vi "Read Name.vi"(8 "error in (no error)":errorcluster, 11 "Player in":refnum<class "Player.lvclass">) -> (0 "error out":errorcluster, 2 "Name":u16(ring) items=["玩家1", "玩家2"], 3 "Player out":refnum<class "Player.lvclass">)   [LabVIEW 2009, in "Player.lvclass"]
doc: "Get the name of the current player."
uses:
  Player.lvclass
  Player.lvclass/Player.ctl
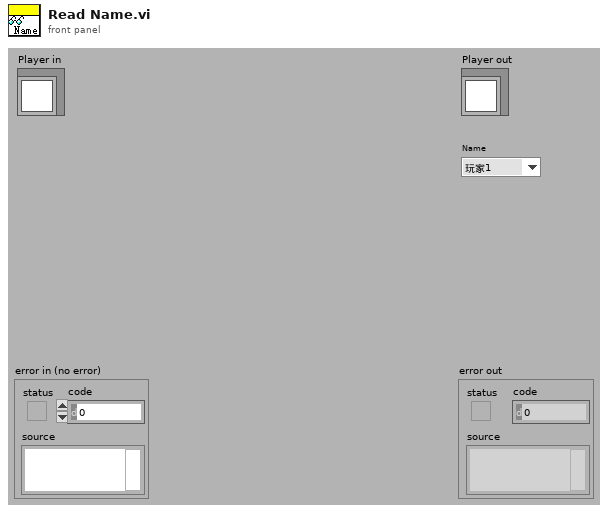
[diagram p1: front panel]
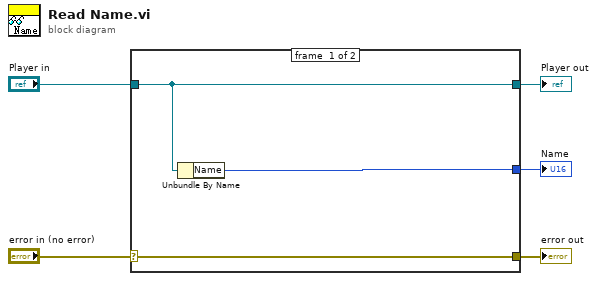
[diagram p0: block diagram]
diagram:
  n1 = case shown="No Error" "error in (no error)" {
    selector: "error in (no error)" -> [w8 w9]
    tunnel: [w8 w9] -> w4
    tunnel: [w7 w10] -> w2
    tunnel: "Player in" -> [w7 w10]
    tunnel: [w6 _] -> w1
    frame #0 {
      n2 = Unbundle By Name(w7) -> ("Name"=w6:u16)
    }
    frame #1 {
    }
  }
  "error out" <- w4
  "Player out" <- w2
  "Name" <- w1
